vi "array.vi"() -> ()   [LabVIEW 2017]
panel:
  out "Array 2":string[](array[string])
  in  "Array":string[](array[string])
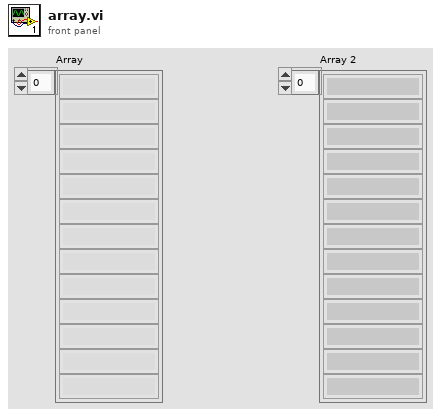
[diagram p1: front panel]
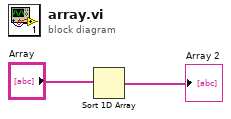
[diagram p0: block diagram]
diagram:
  n1 = Sort 1D Array(array="Array") -> (sorted array=→"Array 2":string[])
